vi "Insight_RW_Beginning_Wavelength.vi"(6 "Atlas Version":T1, 7 "Parameter Type":enum16{"Value", "MAXimum", "MINimum", "DEFault"}(ring), 8 "error in (no error)":errorcluster, 9 "Mode (Read / Write)":enum8{"Write", "Read"}(ring), 10 "Beginning Wavelength (nm)":dbl=1520.0 format="%.4g", 11 "telnet connection":T2) -> (0 "error out":errorcluster, 1 "response data":string, 2 "Beginning Wavelength (nm)":dbl format="%.4g", 3 "telnet  connection out":T2)   [LabVIEW 2015]
doc: "Insight Photonic Solutions\n\nThis VI reads or writes the Minimum Wavelength of the laser sweep. The minimum wavelength is the beginning wavelength if the sweep direction is Increasing Wavelength.\n\nINPUTS\n\nMode - Tells the VI whether the command is a Read or a Write. (Default = Read).\nParameter Type - Tells the VI whether the command should use a Value or a keyword MAXimum, MINimum or DEFault to set the parameter value. (Default = Value).\nBeginning Wavelength (nm) - The numeric value to set the minimum wavelength of a sweep. (Default = 1550).\nAtlas Version - cluster containing the Major, Minor and Build number of the Atlas laser software. This may determine the form of the command used to read/write to the laser.\nerror in - The standard LabView Error cluster. Use this to enforce sequentiality and error tracking.\n\nOUTPUTS\n\nresponse data - the complete response string from the laser\nBeginning Wavelength (nm) - the minimum wavelength of the sweep that is written to or read from the laser\nerror out - the standard error cluster. Reports errors in reading or writing to the laser, or passes through errors from before this VI.\n\nver 1.0 - original release\nver 1.2 - adds parser handling for responses from Atlas version 3.1 or earlier, or version 3.2\nver 3.4 - accepts key word values Max, Min or Default in addition to numeric values of the parameter\nver 3.5 - uses the Atlas Version cluster to distinguish between :CONFigure:SWEep:BWAVelength form of the command and the newer form, :CONFigure:SWEep:WMINimum. This terminology provides more information for bidirectional sweeping."
uses:
  Telnet Session.ctl
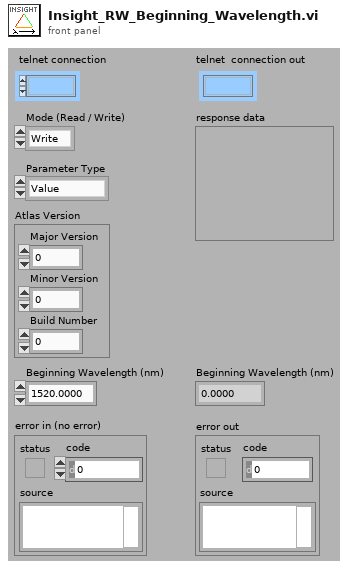
[diagram p1: front panel]
types:
  T1 = cluster{"Major Version":u32, "Minor Version":u32, "Build Number":u32}
  T2 = typedef "Telnet Session.ctl" = refnum<k1>
  T3 = enum16{"Main", "Main, Minor", "Main, Minor, Build"}
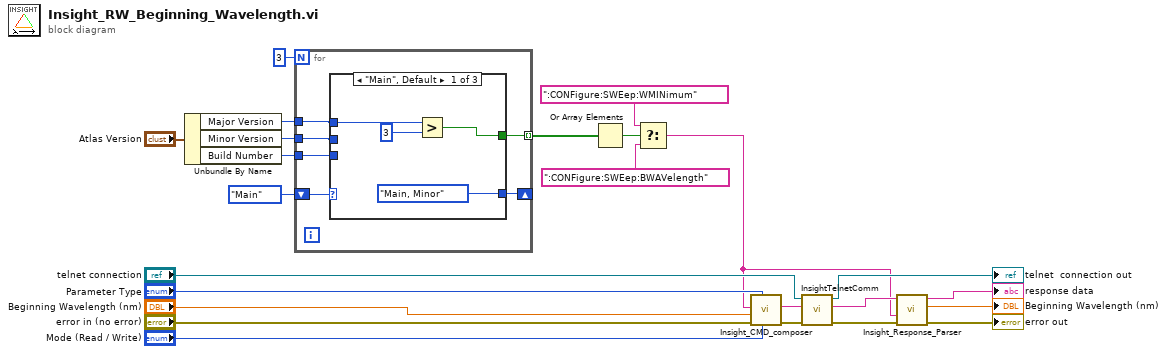
[diagram p0: block diagram]
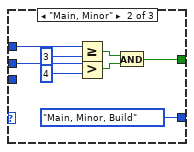
[diagram p2: hidden frame]
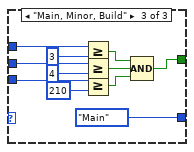
[diagram p3: hidden frame]
diagram:
  n1 = Unbundle By Name("Atlas Version") -> ("Major Version"=w8:u32, "Minor Version"=w7:u32, "Build Number"=w6:u32)
  n2 = for {
    N: 3 -> [_]
    tunnel: w8 -> [w29]
    tunnel: w7 -> [w28]
    tunnel: w6 -> [w27]
    shift-right: [w26] -> _
    shift-left: T3."Main" -> [w30]
    tunnel: [w25] -> w4 mode=indexing
    n3 = case shown="\"Main\", Default" w30 {
      tunnel: [w33 w36 w44] -> w25
      tunnel: w28 -> [_ w38 w49]
      tunnel: w29 -> [w32 w37 w50]
      tunnel: w27 -> [_ _ w48]
      tunnel: [T3."Main, Minor" T3."Main, Minor, Build" T3."Main"] -> w26
      frame "Main", Default {
        n4 = Greater?(x=w32, y=u32 3) -> (0:w33:bool)
      }
      frame "Main, Minor" {
        n5 = Greater Or Equal?(x=w37, y=u32 3) -> (x >= y?=w40:bool)
        n6 = Greater?(x=w38, y=u32 4) -> (0:w39:bool)
        n7 = And(x=w40, y=w39) -> (x .and. y?=w36:bool)
      }
      frame "Main, Minor, Build" {
        n8 = Greater Or Equal?(x=w50, y=u32 3) -> (x >= y?=w47:bool)
        n9 = Greater Or Equal?(x=w49, y=u32 4) -> (x >= y?=w46:bool)
        n10 = Greater Or Equal?(x=w48, y=u32 210) -> (x >= y?=w45:bool)
        n11 = Compound Arithmetic op=AND(w47, w46, w45) -> (w44:bool)
      }
    }
  }
  n12 = Or Array Elements(Boolean array=w4) -> (logical OR=w3:bool)
  n13 = Select(t=":CONFigure:SWEep:WMINimum" ("String"), s=w3, f=":CONFigure:SWEep:BWAVelength" ("String")) -> (s? t:f=w1:string)
  n14 = call "Insight_CMD_composer.vi"("Mode (Read / Write)"="Mode (Read / Write)", "Parameter Type"="Parameter Type", "error in (no error)"="error in (no error)", "Value"="Beginning Wavelength (nm)", "CMD"=w1) -> ("error out"=w22:errorcluster, "Command String"=w18:string)  [unwired: 5 in]
  n15 = call "InsightTelnetComm.vi"("error in"=w22, "write buffer (\"\")"=w18, "telnet connection"="telnet connection") -> ("error out"=w16:errorcluster, "response data"=w15:string, "telnet  connection out"=→"telnet  connection out":T2)  [unwired: 4 in]
  n16 = call "Insight_Response_Parser.vi"("error in (no error)"=w16, "Command String"=w1, "Laser Response In"=w15) -> ("error out"=→"error out":errorcluster, "Value"=→"Beginning Wavelength (nm)":dbl, "Laser Response Out"=→"response data":string)  [unwired: 6 in]
